vi "Insts_init.vi"(2 "Initialize sweep instruments ??":u64[](array[numeric]), 3 "sweep_list":string[](array[string])=["0:0"], 4 "Initialize readout instruments??":u64[](array[numeric]), 5 "Inst_array":T2(array[cluster])) -> (0 "Sweep inst parameters":T1(array[cluster]), 1 "Readout inst parameters":T1(array[cluster]))   [LabVIEW 2013]
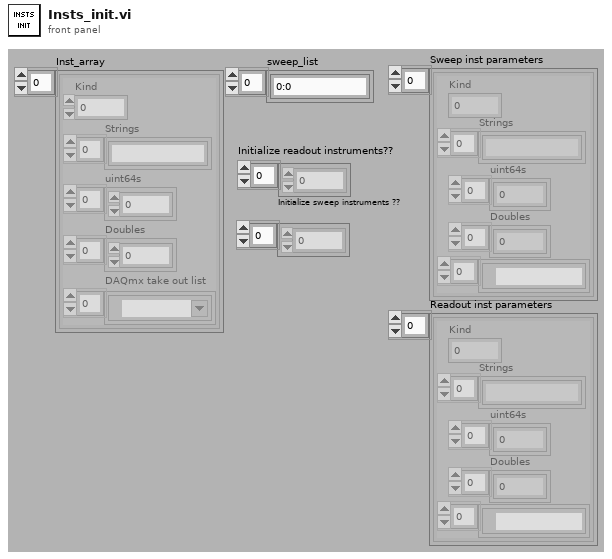
[diagram p1: front panel]
types:
  T1 = cluster{"Kind":u16, "Strings":string[], "uint64s":u64[], "Doubles":dbl[], refnum<k21>[]}[]
  T2 = cluster{"Kind":u16, "Strings":string[], "uint64s":u64[], "Doubles":dbl[], "DAQmx take out list":refnum<k21>[]}[]
  T3 = cluster{"Kind":u16, "Strings":string[], "uint64s":u64[], "Doubles":dbl[], refnum<k21>[]}
  T4 = cluster{"Kind":u16, "Strings":string[], "uint64s":u64[], "Doubles":dbl[], "DAQmx take out list":refnum<k21>[]}
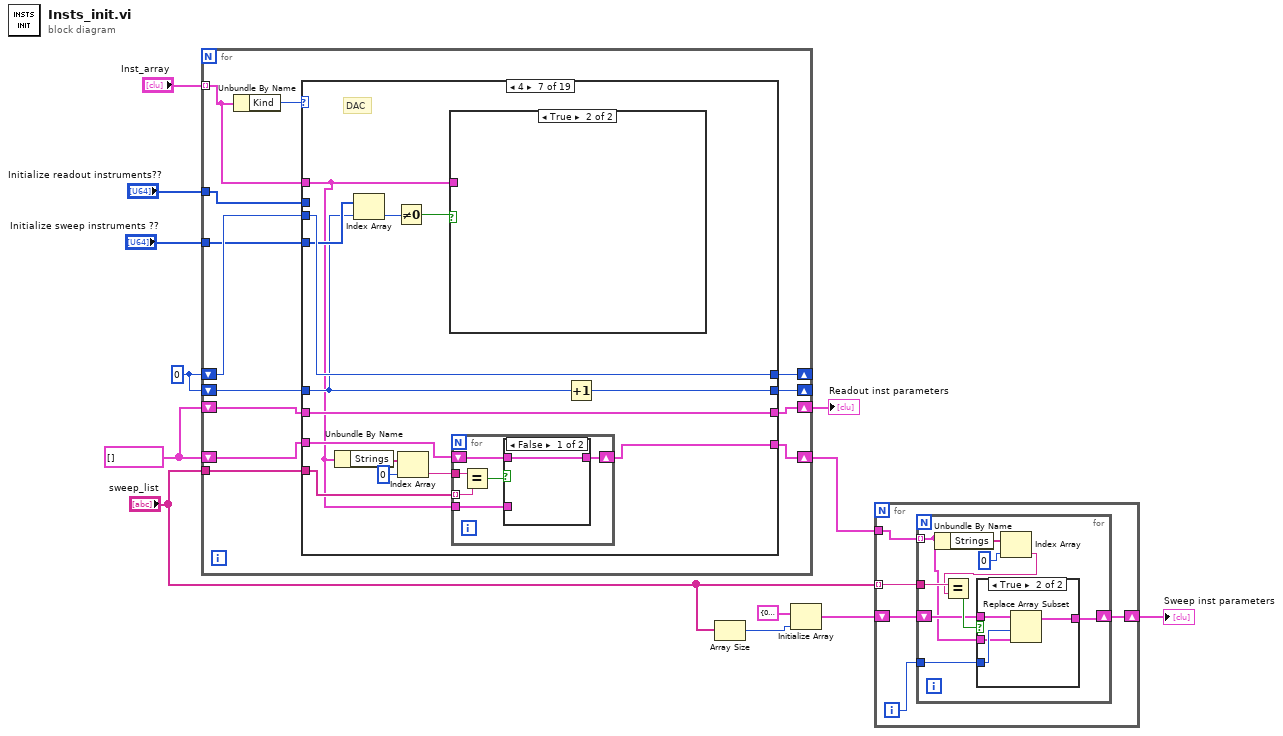
[diagram p0: block diagram]
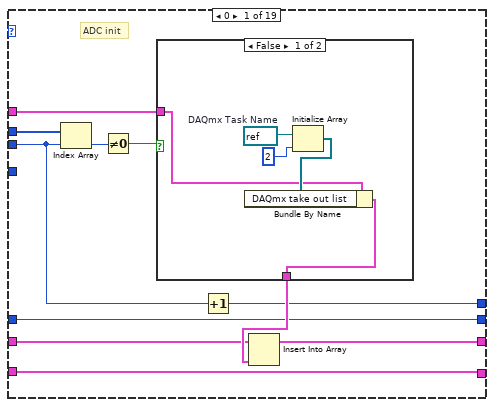
[diagram p3: hidden frame]
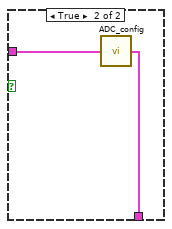
[diagram p4: hidden frame]
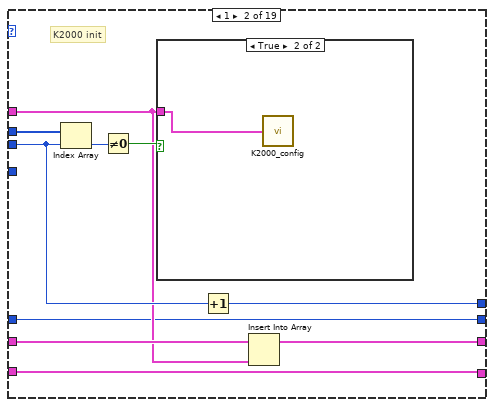
[diagram p5: hidden frame]
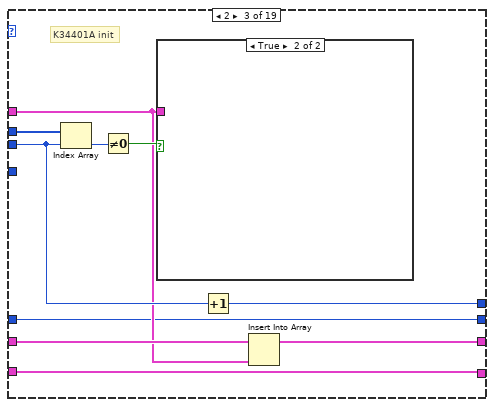
[diagram p7: hidden frame]
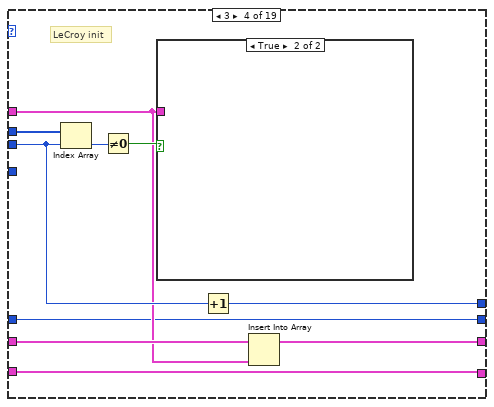
[diagram p9: hidden frame]
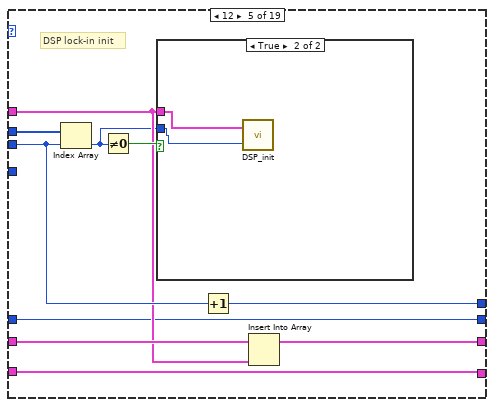
[diagram p11: hidden frame]
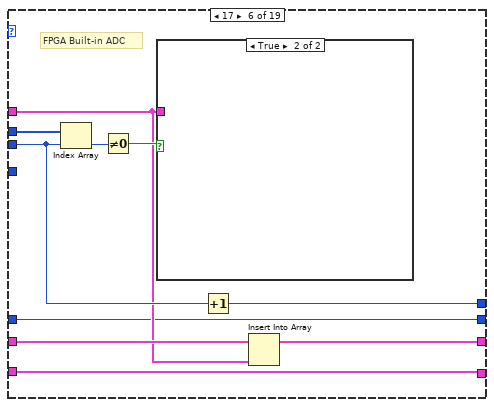
[diagram p13: hidden frame]
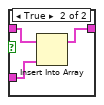
[diagram p15: hidden frame]
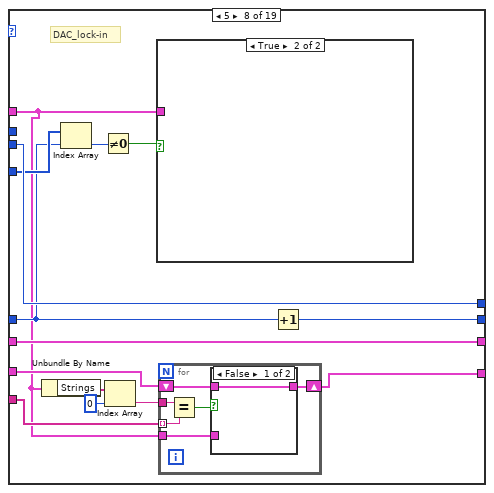
[diagram p17: hidden frame]
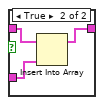
[diagram p18: hidden frame]
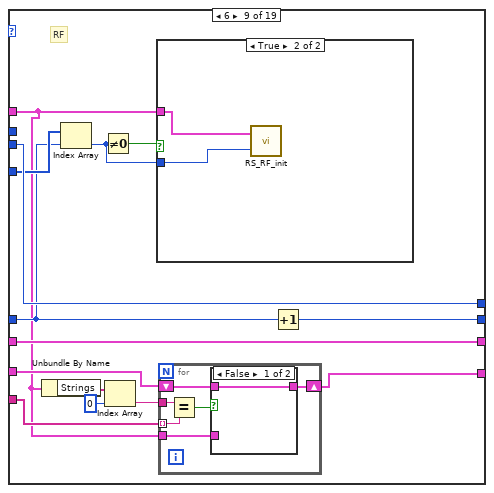
[diagram p20: hidden frame]
diagram:
  w9 = 0
  w8 = T1 [] ("Readout parameters")
  n1 = for {
    tunnel: "Inst_array" -> [w22] mode=indexing
    tunnel: "Initialize sweep instruments ??" -> [w19]
    tunnel: "Initialize readout instruments??" -> [w23]
    shift-right: [w13] -> w7
    shift-left: w8 -> [w16]
    shift-right: [w14] -> w2
    shift-left: w8 -> [w15]
    shift-right: [w21] -> _
    shift-left: w9 -> [w24]
    shift-right: [w18] -> _
    shift-left: w9 -> [w20]
    tunnel: "sweep_list" -> [w17]
    n2 = Unbundle By Name(w22) -> ("Kind"=w25:u16)
    n3 = case shown="4" w25 {
      tunnel: w24 -> [w31 w50 w61 w71 w82 w94 w108 w132 w157 w183 w209 w233 w257 w281 w305 w329 w353 w379 w396]
      tunnel: w23 -> [w36 w53 w64 w74 w84 w96 _ _ _ _ _ _ _ _ _ _ _ _ _]
      tunnel: w22 -> [w33 w46 w57 w67 w78 w90 w97 w121 w146 w172 w198 w222 w246 w270 w294 w318 w342 w368 _]
      tunnel: [w30 w49 w60 w70 w81 w93 w108 w132 w157 w183 w209 w233 w257 w281 w305 w329 w353 w379 w396] -> w21
      tunnel: w16 -> [w29 w48 w59 w69 w80 w92 w105 w129 w154 w180 w206 w230 w254 w278 w302 w326 w350 w376 w395]
      tunnel: [w28 w47 w58 w68 w79 w91 w105 w129 w154 w180 w206 w230 w254 w278 w302 w326 w350 w376 w395] -> w13
      tunnel: w20 -> [w27 w45 w56 w66 w77 w89 w104 w128 w153 w179 w205 w229 w253 w277 w301 w325 w349 w375 w394]
      tunnel: w19 -> [_ _ _ _ _ _ w107 w131 w156 w182 w208 w232 w256 w280 w304 w328 w352 w378 _]
      tunnel: [w27 w45 w56 w66 w77 w89 w106 w130 w155 w181 w207 w231 w255 w279 w303 w327 w351 w377 w394] -> w18
      tunnel: w15 -> [w26 w44 w55 w65 w76 w88 w99 w123 w148 w174 w200 w224 w248 w272 w296 w320 w344 w370 w393]
      tunnel: [w26 w44 w55 w65 w76 w88 w98 w122 w147 w173 w199 w223 w247 w271 w295 w319 w343 w369 w393] -> w14
      tunnel: w17 -> [_ _ _ _ _ _ w100 w124 w149 w175 w201 w225 w249 w273 w297 w321 w345 w371 _]
      frame 0 {
        # "ADC init"
        n4 = Index Array(array=w36, index=w31) -> (element=w35:u64)
        n5 = Not Equal To 0?(x=w35) -> (x != 0?=w34:bool)
        n6 = case shown="False" w34 {
          tunnel: w33 -> [w38 w43]
          tunnel: [w37 w42] -> w32
          frame False {
            w41 = refnum<k21> refnum  # DAQmx Task Name
            n7 = Initialize Array(w41, 2) -> (w39:refnum<k21>[])
            n8 = Bundle By Name(cluster=w38, "DAQmx take out list"=w39) -> (w37:T4)
          }
          frame True {
            n9 = call "ADC_config.vi"("Inst_parameter"=w43) -> ("Inst_parameter out"=w42:T4)
          }
        }
        n10 = Increment(x=w31) -> (x+1=w30:i32)
        n11 = Insert Into Array(array=w29, new element=w32) -> (w28:T1)  [unwired: 1 in]
      }
      frame 1 {
        # "K2000 init"
        n12 = Index Array(array=w53, index=w50) -> (element=w52:u64)
        n13 = Not Equal To 0?(x=w52) -> (x != 0?=w51:bool)
        n14 = case shown="True" w51 {
          tunnel: w46 -> [_ w54]
          frame False {
          }
          frame True {
            n15 = call "K2000_config.vi"("Readout_inst_parameters"=w54) -> ()  [unwired: 1 out]
          }
        }
        n16 = Increment(x=w50) -> (x+1=w49:i32)
        n17 = Insert Into Array(array=w48, new element=w46) -> (w47:T1)  [unwired: 1 in]
      }
      frame 2 {
        # "K34401A init"
        n18 = Index Array(array=w64, index=w61) -> (element=w63:u64)
        n19 = Not Equal To 0?(x=w63) -> (x != 0?=w62:bool)
        n20 = case shown="True" w62 {
          tunnel: w57 -> [_ _]
          frame False {
          }
          frame True {
          }
        }
        n21 = Increment(x=w61) -> (x+1=w60:i32)
        n22 = Insert Into Array(array=w59, new element=w57) -> (w58:T1)  [unwired: 1 in]
      }
      frame 3 {
        # "LeCroy init"
        n23 = Index Array(array=w74, index=w71) -> (element=w73:u64)
        n24 = Not Equal To 0?(x=w73) -> (x != 0?=w72:bool)
        n25 = case shown="True" w72 {
          tunnel: w67 -> [_ _]
          frame False {
          }
          frame True {
          }
        }
        n26 = Increment(x=w71) -> (x+1=w70:i32)
        n27 = Insert Into Array(array=w69, new element=w67) -> (w68:T1)  [unwired: 1 in]
      }
      frame 12 {
        # "DSP lock-in init"
        n28 = Index Array(array=w84, index=w82) -> (element=w75:u64)
        n29 = Not Equal To 0?(x=w75) -> (x != 0?=w83:bool)
        n30 = case shown="True" w83 {
          tunnel: w78 -> [_ w86]
          tunnel: w75 -> [_ w85]
          frame False {
          }
          frame True {
            n31 = call "DSP_init.vi"("Initialize Instrument"=w85, "Inst_param"=w86) -> ()  [unwired: 1 in]
          }
        }
        n32 = Increment(x=w82) -> (x+1=w81:i32)
        n33 = Insert Into Array(array=w80, new element=w78) -> (w79:T1)  [unwired: 1 in]
      }
      frame 17 {
        # "FPGA Built-in ADC"
        n34 = Index Array(array=w96, index=w94) -> (element=w87:u64)
        n35 = Not Equal To 0?(x=w87) -> (x != 0?=w95:bool)
        n36 = case shown="True" w95 {
          tunnel: w90 -> [_ _]
          frame False {
          }
          frame True {
          }
        }
        n37 = Increment(x=w94) -> (x+1=w93:i32)
        n38 = Insert Into Array(array=w92, new element=w90) -> (w91:T1)  [unwired: 1 in]
      }
      frame 4 {
        # "DAC"
        n39 = Unbundle By Name(w97) -> ("Strings"=w103:string[])
        n40 = Index Array(array=w107, index=w104) -> (element=w110:u64)
        n41 = Not Equal To 0?(x=w110) -> (x != 0?=w109:bool)
        n42 = Index Array(array=w103, index=0) -> (element=w101:string)
        n43 = case shown="True" w109 {
          tunnel: w97 -> [_ _]
          frame False {
          }
          frame True {
          }
        }
        n44 = for {
          tunnel: w101 -> [w116]
          tunnel: w100 -> [w115] mode=indexing
          shift-right: [w111] -> w98
          shift-left: w99 -> [w112]
          tunnel: w97 -> [w113]
          n45 = Equal?(x=w116, y=w115) -> (x = y?=w114:bool)
          n46 = case shown="False" w114 {
            tunnel: w113 -> [_ w120]
            tunnel: w112 -> [w117 w119]
            tunnel: [w117 w118] -> w111
            frame False {
            }
            frame True {
              n47 = Insert Into Array(array=w119, new element=w120) -> (w118:T1)  [unwired: 1 in]
            }
          }
        }
        n48 = Increment(x=w104) -> (x+1=w106:i32)
      }
      frame 5 {
        # "DAC_lock-in"
        n49 = Unbundle By Name(w121) -> ("Strings"=w127:string[])
        n50 = Index Array(array=w131, index=w128) -> (element=w134:u64)
        n51 = Not Equal To 0?(x=w134) -> (x != 0?=w133:bool)
        n52 = Index Array(array=w127, index=0) -> (element=w125:string)
        n53 = case shown="True" w133 {
          tunnel: w121 -> [_ _]
          frame False {
          }
          frame True {
          }
        }
        n54 = for {
          tunnel: w125 -> [w140]
          tunnel: w124 -> [w139] mode=indexing
          shift-right: [w135] -> w122
          shift-left: w123 -> [w136]
          tunnel: w121 -> [w137]
          n55 = Equal?(x=w140, y=w139) -> (x = y?=w138:bool)
          n56 = case shown="False" w138 {
            tunnel: w137 -> [_ w144]
            tunnel: w136 -> [w141 w143]
            tunnel: [w141 w142] -> w135
            frame False {
            }
            frame True {
              n57 = Insert Into Array(array=w143, new element=w144) -> (w142:T1)  [unwired: 1 in]
            }
          }
        }
        n58 = Increment(x=w128) -> (x+1=w130:i32)
      }
      frame 6 {
        # "RF"
        n59 = Unbundle By Name(w146) -> ("Strings"=w152:string[])
        n60 = Index Array(array=w156, index=w153) -> (element=w145:u64)
        n61 = Not Equal To 0?(x=w145) -> (x != 0?=w158:bool)
        n62 = Index Array(array=w152, index=0) -> (element=w150:string)
        n63 = case shown="True" w158 {
          tunnel: w146 -> [_ w170]
          tunnel: w145 -> [_ w169]
          frame False {
          }
          frame True {
            n64 = call "RS_RF_init.vi"("Initialize Instrument"=w169, "Inst_param"=w170) -> ()  [unwired: 1 in]
          }
        }
        n65 = for {
          tunnel: w150 -> [w164]
          tunnel: w149 -> [w163] mode=indexing
          shift-right: [w159] -> w147
          shift-left: w148 -> [w160]
          tunnel: w146 -> [w161]
          n66 = Equal?(x=w164, y=w163) -> (x = y?=w162:bool)
          n67 = case shown="False" w162 {
            tunnel: w161 -> [_ w168]
            tunnel: w160 -> [w165 w167]
            tunnel: [w165 w166] -> w159
            frame False {
            }
            frame True {
              n68 = Insert Into Array(array=w167, new element=w168) -> (w166:T1)  [unwired: 1 in]
            }
          }
        }
        n69 = Increment(x=w153) -> (x+1=w155:i32)
      }
      frame 7 {
        # "AWG"
        n70 = Unbundle By Name(w172) -> ("Strings"=w178:string[])
        n71 = Index Array(array=w182, index=w179) -> (element=w171:u64)
        n72 = Not Equal To 0?(x=w171) -> (x != 0?=w184:bool)
        n73 = Index Array(array=w178, index=0) -> (element=w176:string)
        n74 = case shown="True" w184 {
          tunnel: w172 -> [_ w196]
          tunnel: w171 -> [_ w195]
          frame False {
          }
          frame True {
            n75 = call "AWG_init.vi"("Initialize?"=w195, "Inst_param"=w196) -> ()  [unwired: 1 out]
          }
        }
        n76 = for {
          tunnel: w176 -> [w190]
          tunnel: w175 -> [w189] mode=indexing
          shift-right: [w185] -> w173
          shift-left: w174 -> [w186]
          tunnel: w172 -> [w187]
          n77 = Equal?(x=w190, y=w189) -> (x = y?=w188:bool)
          n78 = case shown="False" w188 {
            tunnel: w187 -> [_ w194]
            tunnel: w186 -> [w191 w193]
            tunnel: [w191 w192] -> w185
            frame False {
            }
            frame True {
              n79 = Insert Into Array(array=w193, new element=w194) -> (w192:T1)  [unwired: 1 in]
            }
          }
        }
        n80 = Increment(x=w179) -> (x+1=w181:i32)
      }
      frame 8 {
        # "B-field"
        n81 = Unbundle By Name(w198) -> ("Strings"=w204:string[])
        n82 = Index Array(array=w208, index=w205) -> (element=w197:u64)
        n83 = Not Equal To 0?(x=w197) -> (x != 0?=w210:bool)
        n84 = Index Array(array=w204, index=0) -> (element=w202:string)
        n85 = case shown="True" w210 {
          tunnel: w198 -> [_ _]
          tunnel: w197 -> [_ _]
          frame False {
          }
          frame True {
          }
        }
        n86 = for {
          tunnel: w202 -> [w216]
          tunnel: w201 -> [w215] mode=indexing
          shift-right: [w211] -> w199
          shift-left: w200 -> [w212]
          tunnel: w198 -> [w213]
          n87 = Equal?(x=w216, y=w215) -> (x = y?=w214:bool)
          n88 = case shown="False" w214 {
            tunnel: w213 -> [_ w220]
            tunnel: w212 -> [w217 w219]
            tunnel: [w217 w218] -> w211
            frame False {
            }
            frame True {
              n89 = Insert Into Array(array=w219, new element=w220) -> (w218:T1)  [unwired: 1 in]
            }
          }
        }
        n90 = Increment(x=w205) -> (x+1=w207:i32)
      }
      frame 9 {
        # "Fast sequence"
        n91 = Unbundle By Name(w222) -> ("Strings"=w228:string[])
        n92 = Index Array(array=w232, index=w229) -> (element=w221:u64)
        n93 = Not Equal To 0?(x=w221) -> (x != 0?=w234:bool)
        n94 = Index Array(array=w228, index=0) -> (element=w226:string)
        n95 = case shown="True" w234 {
          tunnel: w222 -> [_ _]
          tunnel: w221 -> [_ _]
          frame False {
          }
          frame True {
          }
        }
        n96 = for {
          tunnel: w226 -> [w240]
          tunnel: w225 -> [w239] mode=indexing
          shift-right: [w235] -> w223
          shift-left: w224 -> [w236]
          tunnel: w222 -> [w237]
          n97 = Equal?(x=w240, y=w239) -> (x = y?=w238:bool)
          n98 = case shown="False" w238 {
            tunnel: w237 -> [_ w244]
            tunnel: w236 -> [w241 w243]
            tunnel: [w241 w242] -> w235
            frame False {
            }
            frame True {
              n99 = Insert Into Array(array=w243, new element=w244) -> (w242:T1)  [unwired: 1 in]
            }
          }
        }
        n100 = Increment(x=w229) -> (x+1=w231:i32)
      }
      frame 10 {
        # "Fast sequence slot"
        n101 = Unbundle By Name(w246) -> ("Strings"=w252:string[])
        n102 = Index Array(array=w256, index=w253) -> (element=w245:u64)
        n103 = Not Equal To 0?(x=w245) -> (x != 0?=w258:bool)
        n104 = Index Array(array=w252, index=0) -> (element=w250:string)
        n105 = case shown="True" w258 {
          tunnel: w246 -> [_ _]
          tunnel: w245 -> [_ _]
          frame False {
          }
          frame True {
          }
        }
        n106 = for {
          tunnel: w250 -> [w264]
          tunnel: w249 -> [w263] mode=indexing
          shift-right: [w259] -> w247
          shift-left: w248 -> [w260]
          tunnel: w246 -> [w261]
          n107 = Equal?(x=w264, y=w263) -> (x = y?=w262:bool)
          n108 = case shown="False" w262 {
            tunnel: w261 -> [_ w268]
            tunnel: w260 -> [w265 w267]
            tunnel: [w265 w266] -> w259
            frame False {
            }
            frame True {
              n109 = Insert Into Array(array=w267, new element=w268) -> (w266:T1)  [unwired: 1 in]
            }
          }
        }
        n110 = Increment(x=w253) -> (x+1=w255:i32)
      }
      frame 11 {
        # "Command line"
        n111 = Unbundle By Name(w270) -> ("Strings"=w276:string[])
        n112 = Index Array(array=w280, index=w277) -> (element=w269:u64)
        n113 = Not Equal To 0?(x=w269) -> (x != 0?=w282:bool)
        n114 = Index Array(array=w276, index=0) -> (element=w274:string)
        n115 = case shown="True" w282 {
          tunnel: w270 -> [_ _]
          tunnel: w269 -> [_ _]
          frame False {
          }
          frame True {
          }
        }
        n116 = for {
          tunnel: w274 -> [w288]
          tunnel: w273 -> [w287] mode=indexing
          shift-right: [w283] -> w271
          shift-left: w272 -> [w284]
          tunnel: w270 -> [w285]
          n117 = Equal?(x=w288, y=w287) -> (x = y?=w286:bool)
          n118 = case shown="False" w286 {
            tunnel: w285 -> [_ w292]
            tunnel: w284 -> [w289 w291]
            tunnel: [w289 w290] -> w283
            frame False {
            }
            frame True {
              n119 = Insert Into Array(array=w291, new element=w292) -> (w290:T1)  [unwired: 1 in]
            }
          }
        }
        n120 = Increment(x=w277) -> (x+1=w279:i32)
      }
      frame 13 {
        # "DSP lock-in sweep"
        n121 = Unbundle By Name(w294) -> ("Strings"=w300:string[])
        n122 = Index Array(array=w304, index=w301) -> (element=w293:u64)
        n123 = Not Equal To 0?(x=w293) -> (x != 0?=w306:bool)
        n124 = Index Array(array=w300, index=0) -> (element=w298:string)
        n125 = case shown="True" w306 {
          tunnel: w294 -> [_ _]
          tunnel: w293 -> [_ _]
          frame False {
          }
          frame True {
          }
        }
        n126 = for {
          tunnel: w298 -> [w312]
          tunnel: w297 -> [w311] mode=indexing
          shift-right: [w307] -> w295
          shift-left: w296 -> [w308]
          tunnel: w294 -> [w309]
          n127 = Equal?(x=w312, y=w311) -> (x = y?=w310:bool)
          n128 = case shown="False" w310 {
            tunnel: w309 -> [_ w316]
            tunnel: w308 -> [w313 w315]
            tunnel: [w313 w314] -> w307
            frame False {
            }
            frame True {
              n129 = Insert Into Array(array=w315, new element=w316) -> (w314:T1)  [unwired: 1 in]
            }
          }
        }
        n130 = Increment(x=w301) -> (x+1=w303:i32)
      }
      frame 14 {
        # "ms to wait"
        n131 = Unbundle By Name(w318) -> ("Strings"=w324:string[])
        n132 = Index Array(array=w328, index=w325) -> (element=w317:u64)
        n133 = Not Equal To 0?(x=w317) -> (x != 0?=w330:bool)
        n134 = Index Array(array=w324, index=0) -> (element=w322:string)
        n135 = case shown="True" w330 {
          tunnel: w318 -> [_ _]
          tunnel: w317 -> [_ _]
          frame False {
          }
          frame True {
          }
        }
        n136 = for {
          tunnel: w322 -> [w336]
          tunnel: w321 -> [w335] mode=indexing
          shift-right: [w331] -> w319
          shift-left: w320 -> [w332]
          tunnel: w318 -> [w333]
          n137 = Equal?(x=w336, y=w335) -> (x = y?=w334:bool)
          n138 = case shown="False" w334 {
            tunnel: w333 -> [_ w340]
            tunnel: w332 -> [w337 w339]
            tunnel: [w337 w338] -> w331
            frame False {
            }
            frame True {
              n139 = Insert Into Array(array=w339, new element=w340) -> (w338:T1)  [unwired: 1 in]
            }
          }
        }
        n140 = Increment(x=w325) -> (x+1=w327:i32)
      }
      frame 15 {
        # "ATM delay line"
        n141 = Unbundle By Name(w342) -> ("Strings"=w348:string[])
        n142 = Index Array(array=w352, index=w349) -> (element=w341:u64)
        n143 = Not Equal To 0?(x=w341) -> (x != 0?=w354:bool)
        n144 = Index Array(array=w348, index=0) -> (element=w346:string)
        n145 = case shown="True" w354 {
          tunnel: w342 -> [_ w366]
          tunnel: w341 -> [_ w365]
          frame False {
          }
          frame True {
            n146 = call "DelayLineInit.vi"("Inst bool"=w365, "Inst_param"=w366) -> ()  [unwired: 1 in]
          }
        }
        n147 = for {
          tunnel: w346 -> [w360]
          tunnel: w345 -> [w359] mode=indexing
          shift-right: [w355] -> w343
          shift-left: w344 -> [w356]
          tunnel: w342 -> [w357]
          n148 = Equal?(x=w360, y=w359) -> (x = y?=w358:bool)
          n149 = case shown="False" w358 {
            tunnel: w357 -> [_ w364]
            tunnel: w356 -> [w361 w363]
            tunnel: [w361 w362] -> w355
            frame False {
            }
            frame True {
              n150 = Insert Into Array(array=w363, new element=w364) -> (w362:T1)  [unwired: 1 in]
            }
          }
        }
        n151 = Increment(x=w349) -> (x+1=w351:i32)
      }
      frame 16 {
        # "RF Attn"
        n152 = Unbundle By Name(w368) -> ("Strings"=w374:string[])
        n153 = Index Array(array=w378, index=w375) -> (element=w367:u64)
        n154 = Not Equal To 0?(x=w367) -> (x != 0?=w380:bool)
        n155 = Index Array(array=w374, index=0) -> (element=w372:string)
        n156 = case shown="True" w380 {
          tunnel: w368 -> [_ w392]
          tunnel: w367 -> [_ w391]
          frame False {
          }
          frame True {
            n157 = call "RS_RF_init.vi"("Initialize Instrument"=w391, "Inst_param"=w392) -> ()  [unwired: 1 in]
          }
        }
        n158 = for {
          tunnel: w372 -> [w386]
          tunnel: w371 -> [w385] mode=indexing
          shift-right: [w381] -> w369
          shift-left: w370 -> [w382]
          tunnel: w368 -> [w383]
          n159 = Equal?(x=w386, y=w385) -> (x = y?=w384:bool)
          n160 = case shown="False" w384 {
            tunnel: w383 -> [_ w390]
            tunnel: w382 -> [w387 w389]
            tunnel: [w387 w388] -> w381
            frame False {
            }
            frame True {
              n161 = Insert Into Array(array=w389, new element=w390) -> (w388:T1)  [unwired: 1 in]
            }
          }
        }
        n162 = Increment(x=w375) -> (x+1=w377:i32)
      }
      frame 100, Default {
        # "Else"
      }
    }
  }
  "Readout inst parameters" <- w7
  n163 = Array Size(array="sweep_list") -> (size(s)=w4:i32)
  n164 = Initialize Array(T3 {"Kind"=0, "Strings"=[], "uint64s"=[], "Doubles"=[], []}, w4) -> (w3:T1)
  n165 = for {
    tunnel: "sweep_list" -> [w399] mode=indexing
    tunnel: w2 -> [w398]
    shift-right: [w397] -> w1
    shift-left: w3 -> [w401]
    i -> [w400]
    n166 = for {
      shift-right: [w404] -> w397
      shift-left: w401 -> [w405]
      tunnel: w400 -> [w403]
      tunnel: w399 -> [w408]
      tunnel: w398 -> [w402] mode=indexing
      n167 = Unbundle By Name(w402) -> ("Strings"=w410:string[])
      n168 = Index Array(array=w410, index=0) -> (element=w407:string)
      n169 = Equal?(x=w408, y=w407) -> (x = y?=w406:bool)
      n170 = case shown="True" w406 {
        tunnel: w405 -> [w411 w415]
        tunnel: [w411 w414] -> w404
        tunnel: w403 -> [_ w413]
        tunnel: w402 -> [_ w412]
        frame False {
        }
        frame True {
          n171 = Replace Array Subset(array=w415, new element=w412, index=w413) -> (w414:T1)
        }
      }
    }
  }
  "Sweep inst parameters" <- w1
